vi "OAT Waterfall Plot Indicator.vi"() -> ()   [LabVIEW 2017]
doc: "Uses the Waterfall Plot to display the results of the spectral map as a function of time on a customized waveform graph."
uses:
  <vilib>/addons/Sound and Vibration/Order Analysis/Backward Compatibility/SubVIs/OAT Waterfall Plot.ctl
panel:
  out "Waterfall Plot":T1
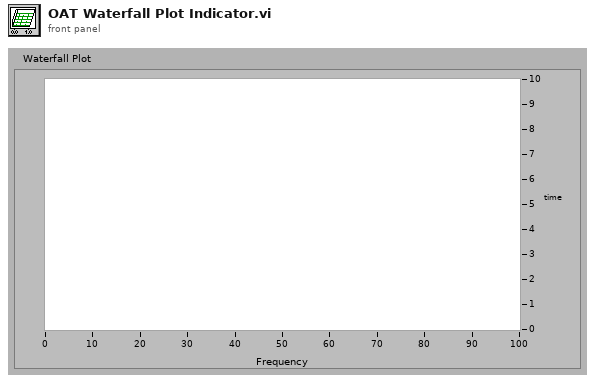
[diagram p1: front panel]
types:
  T1 = typedef "OAT Waterfall Plot.ctl" = cluster{"X0":dbl, "dX":dbl, "Y":dbl[]}[]
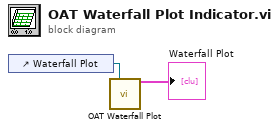
[diagram p0: block diagram]
diagram:
  n1 = control-ref of="Waterfall Plot"() -> (w2:refnum<vi>)
  n2 = call <vilib>:"OAT Waterfall Plot.vi"("waterfall plot ref"=w2) -> ("waterfall plot"=→"Waterfall Plot":T1)  [unwired: 13 in, 1 out]
